vi "PreConfig.vi"(5 "Ruta de Transductores in":path, 7 "Ruta de Mediciones in":path, 8 "error in (no error)":errorcluster, 10 "Transductores":string[][](array[string]), 11 "Medidas":string[][](array[string])) -> (0 "error out":errorcluster, 2 "Transductores":string[][](table), 3 "Mediciones":string[][](array[string]), 4 "Ruta de Transductores Out":path, 6 "Ruta de Mediciones Out":path)   [LabVIEW 2014, in "ConfigProg.lvlib"]
doc: "Carga las Mediciones y los Transducotres."
uses:
  <vilib>/Utility/miscctls.llb/LVPointTypeDef.ctl
  <vilib>/Utility/file.llb/Read From Spreadsheet File (string).vi
  ConfigProg.lvlib
panel:
  in  "Cancel":bool
  in  "Save":bool
  in  "Ruta de Mediciones":path caption="Ruta de Mediciones:"
  in  "Ruta de Transductores":path caption="Ruta de Transductores:"
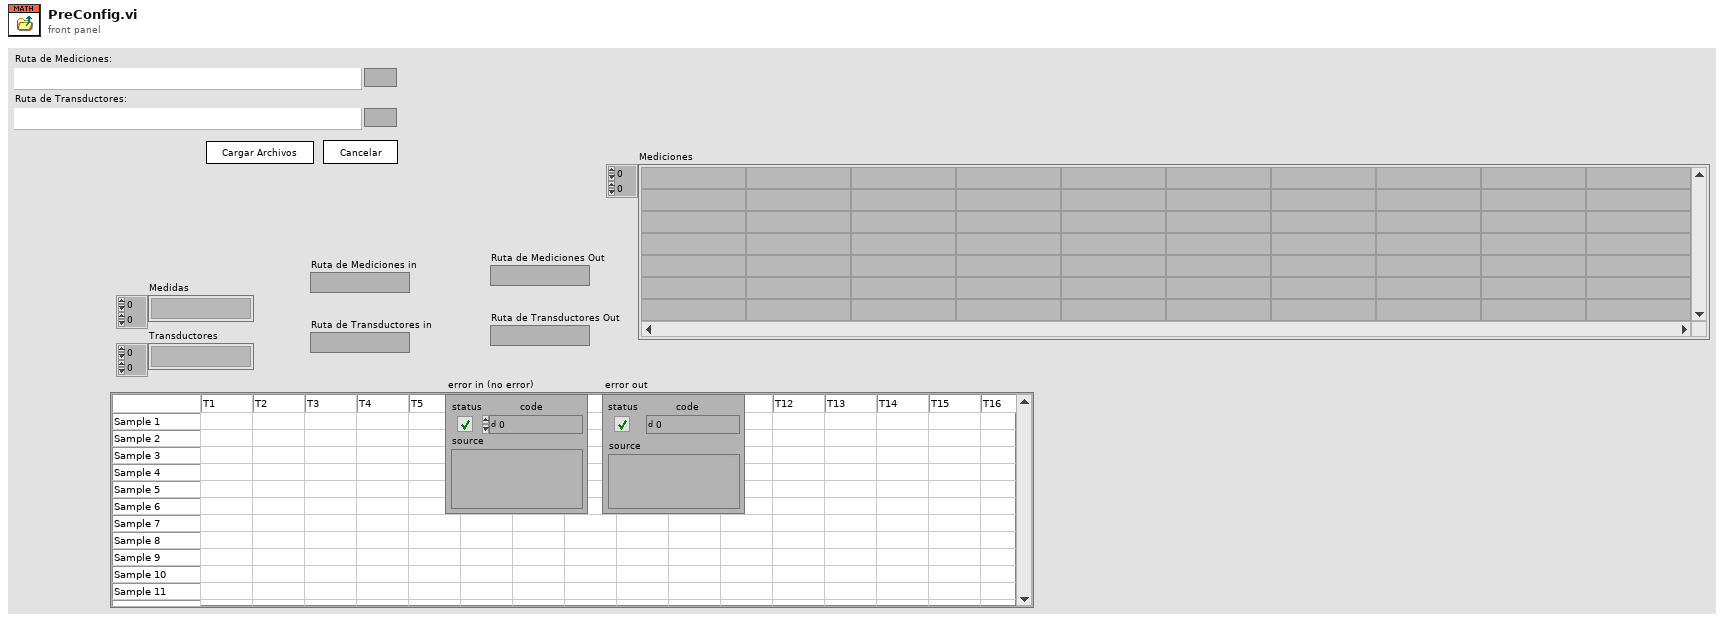
[diagram p1: front panel]
types:
  T1 = typedef "LVPointTypeDef.ctl" = cluster{"Horizontal":i16, "Vertical":i16}
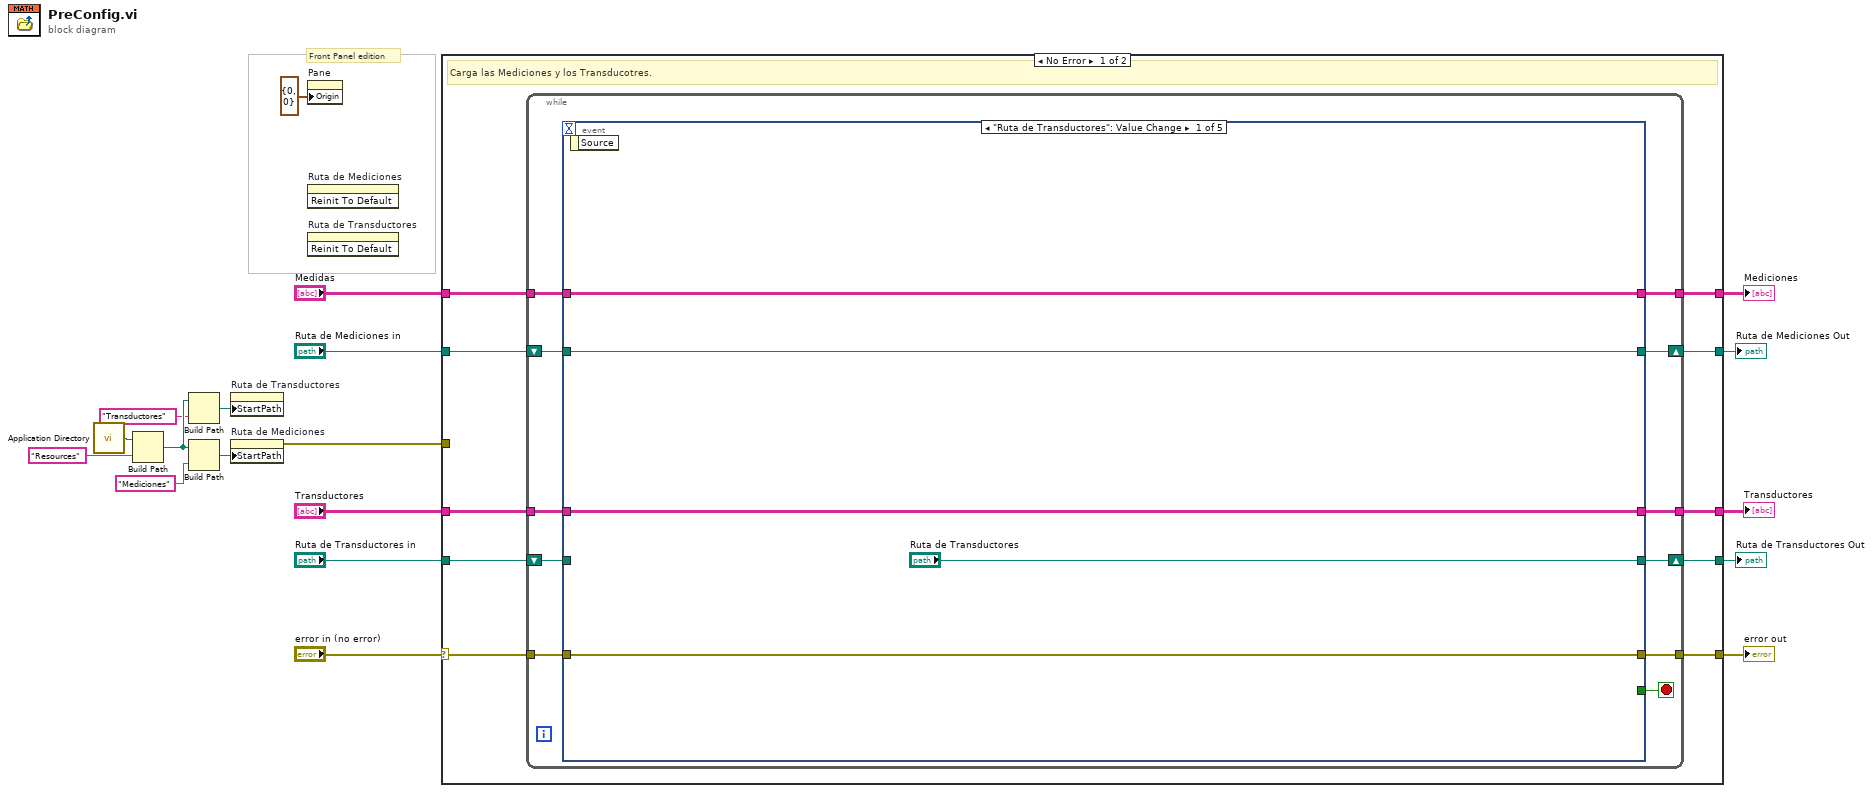
[diagram p0: block diagram]
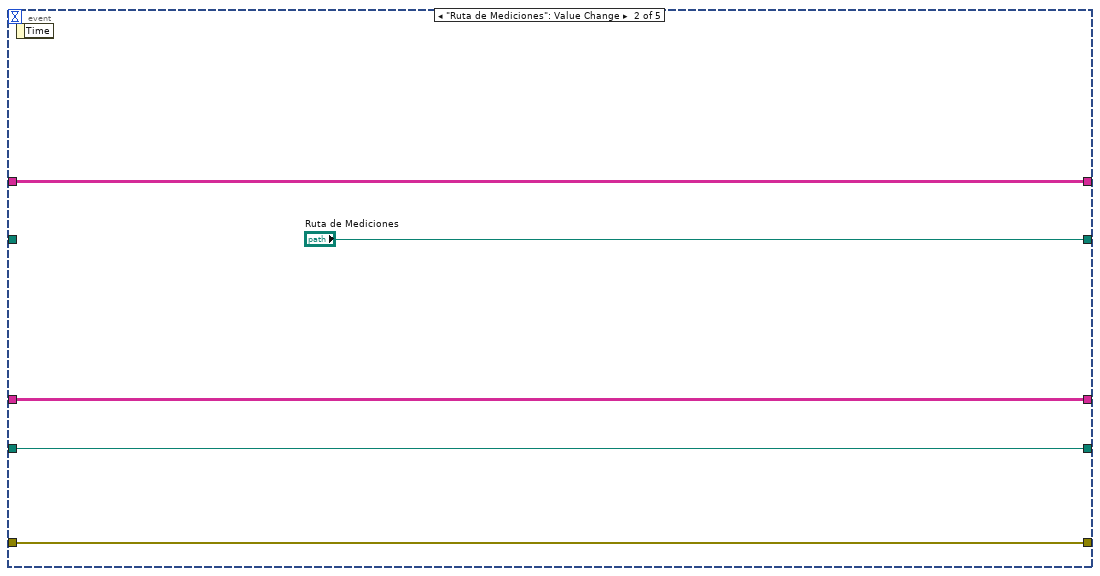
[diagram p2: hidden frame]
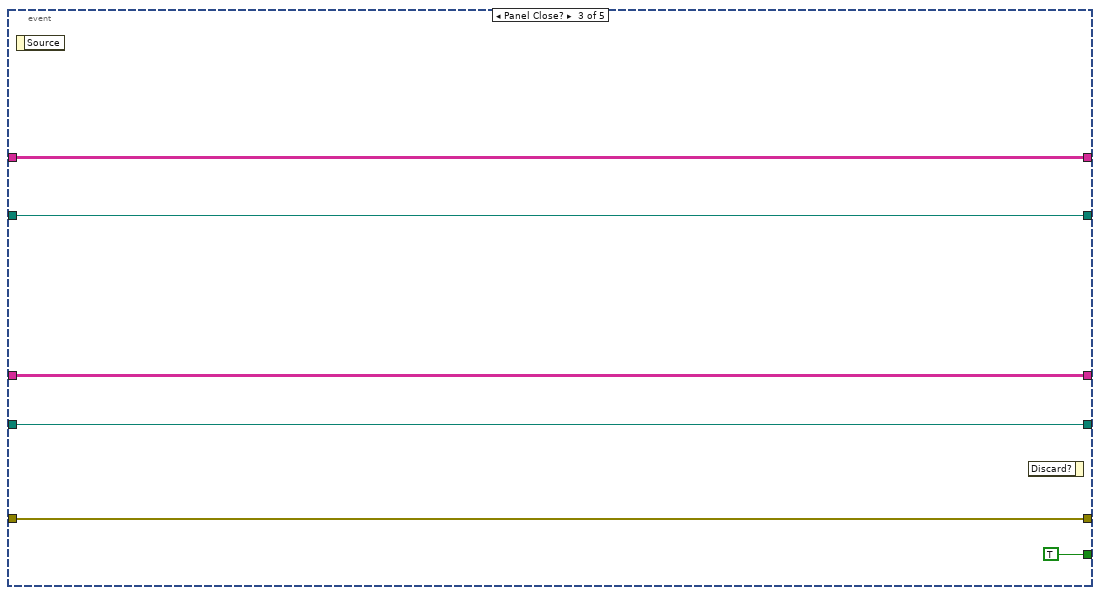
[diagram p3: hidden frame]
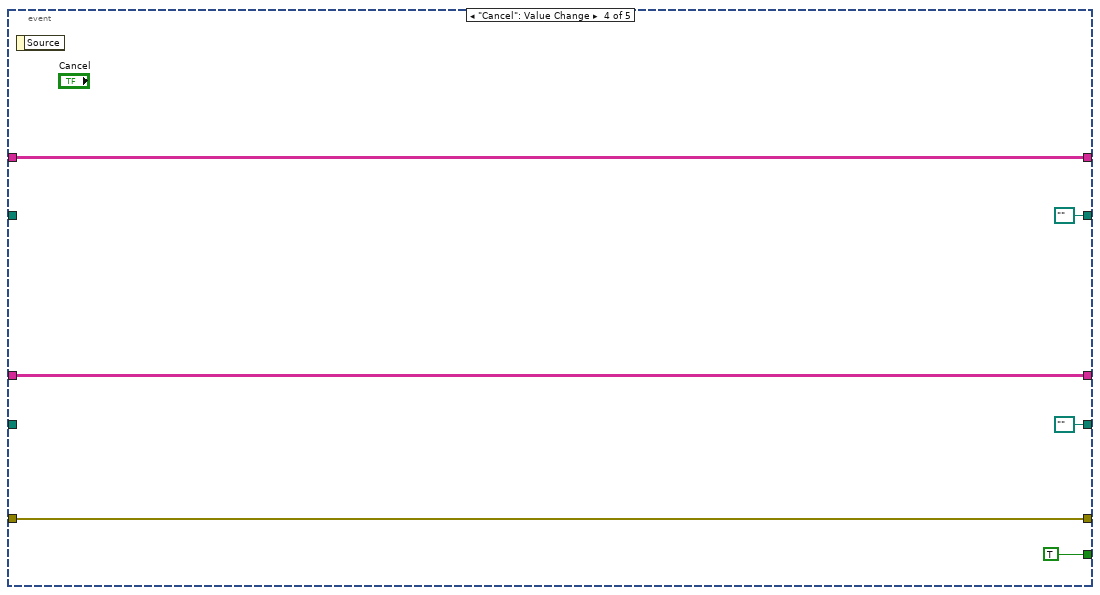
[diagram p4: hidden frame]
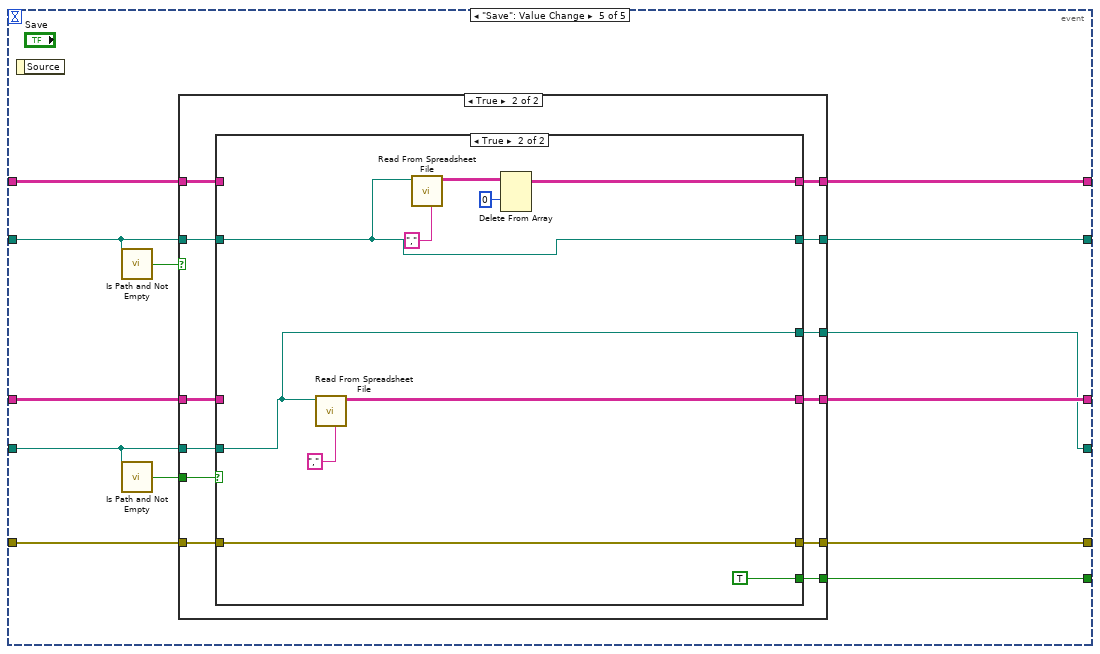
[diagram p5: hidden frame]
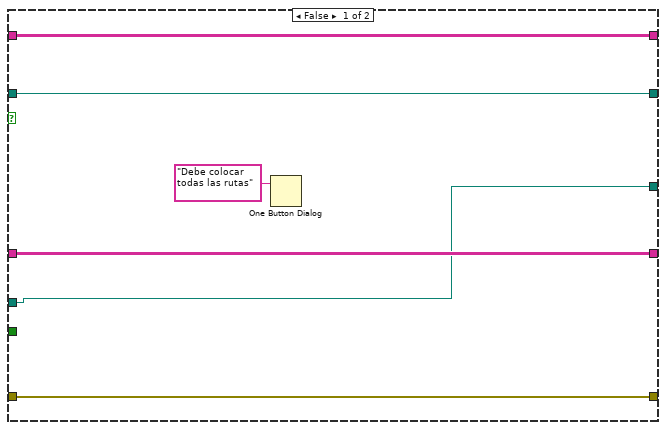
[diagram p6: hidden frame]
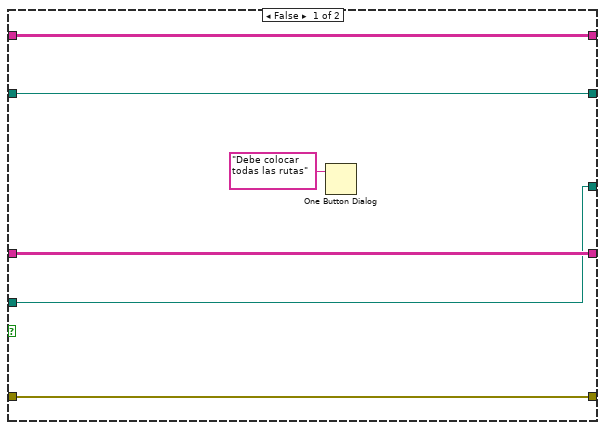
[diagram p7: hidden frame]
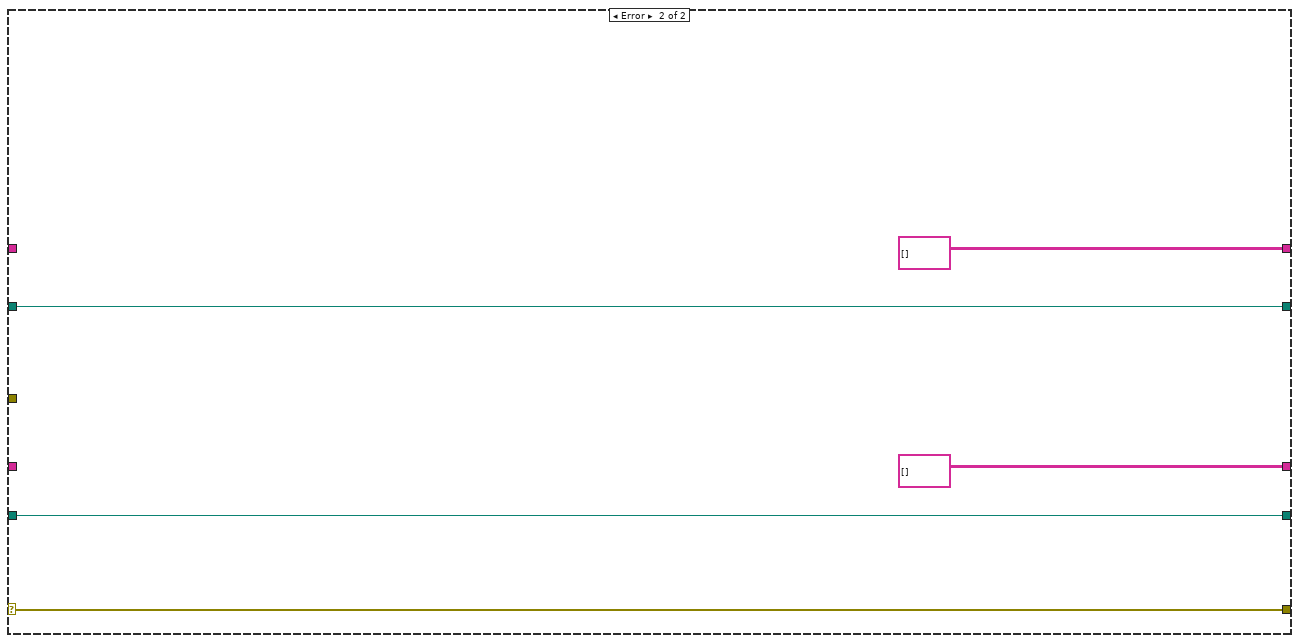
[diagram p8: hidden frame]
diagram:
  # "Front Panel edition"
  n1 = call <vilib>:"Application Directory.vi"() -> ("Application Directory"=w7:path)
  n2 = Build Path(base path=w7, name or relative path="Resources") -> (appended path=w6:path)
  n3 = Build Path(base path=w6, name or relative path="Transductores") -> (appended path=w3:path)
  n4 = Build Path(base path=w6, name or relative path="Mediciones") -> (appended path=w2:path)
  n5 = property on="Ruta de Transductores" class="Path"("StartPath"=w3) -> ()  [unwired: 2 in, 2 out]
  n6 = property on="Ruta de Mediciones" class="Path"("StartPath"=w2) -> (error out=w1:errorcluster)  [unwired: 2 in, 1 out]
  n7 = property on="Pane" class="Pane"("Origin"=T1 {"Horizontal"=0, "Vertical"=0}) -> ()  [unwired: 2 in, 2 out]
  n8 = invoke on="Ruta de Mediciones" class="Path" method="Reinit To Default"() -> ()  [unwired: 3 in, 3 out]
  n9 = invoke on="Ruta de Transductores" class="Path" method="Reinit To Default"() -> ()  [unwired: 3 in, 3 out]
  n10 = case shown="No Error" "error in (no error)" {
    selector: "error in (no error)" -> [w28 w114]
    tunnel: [w29 w114] -> w18
    tunnel: [w26 string[][] []] -> w16
    tunnel: [w27 string[][] []] -> w15
    tunnel: "Medidas" -> [w25 _]
    tunnel: "Transductores" -> [w24 _]
    tunnel: [w23 w111] -> w12
    tunnel: [w22 w110] -> w11
    tunnel: "Ruta de Mediciones in" -> [w21 w111]
    tunnel: "Ruta de Transductores in" -> [w20 w110]
    tunnel: w1 -> [_ _]
    frame No Error {
      # "Carga las Mediciones y los Transducotres."
      n11 = while {
        tunnel: w28 -> [w39]
        tunnel: [w40] -> w29
        shift-right: [w35] -> w22
        shift-left: w20 -> [w33]
        tunnel: [w34] -> w26
        shift-right: [w31] -> w23
        shift-left: w21 -> [w32]
        tunnel: w25 -> [w36]
        tunnel: [w38] -> w27
        tunnel: w24 -> [w30]
        stop <- w37 stop-if-true
        n12 = event shown="[0] \"Ruta de Transductores\": Value Change" {
          selector: _ -> [_ _ _ _ _]
          dyn-events: _ -> [_ _ _ _ _]
          timeout: _ -> [_ _ _ _ _]
          tunnel: [w41 w46 w51 w59 w75] -> w34
          tunnel: [w43 w50 w55 w61 w70] -> w40
          tunnel: w39 -> [w43 w50 w55 w61 w74]
          tunnel: [w45 w47 w52 w60 w73] -> w38
          tunnel: [_ _ TRUE ("Discard?") TRUE ("Discard?") w65] -> w37
          tunnel: w36 -> [w45 w47 w52 w60 w66]
          tunnel: ["Ruta de Transductores" w49 w53 path "" ("Ruta de Transductores in") w64] -> w35
          tunnel: w33 -> [_ w49 w53 _ w71]
          tunnel: w32 -> [w42 _ w54 _ w72]
          tunnel: [w42 "Ruta de Mediciones" w54 path "" ("Ruta de Mediciones in") w63] -> w31
          tunnel: w30 -> [w41 w46 w51 w59 w67]
          event "Ruta de Transductores": Value Change {
            n13 = event-data() -> ()  [unwired: 1 in, 1 out]
          }
          event "Ruta de Mediciones": Value Change {
            n14 = event-data() -> ()  [unwired: 1 in, 1 out]
          }
          event Panel Close? {
            n15 = event-data() -> ()  [unwired: 1 in, 1 out]
            n16 = event-data() -> ()  [unwired: 2 in, 1 out]
          }
          event "Cancel": Value Change {
            n17 = event-data() -> ()  [unwired: 1 in, 1 out]
          }
          event "Save": Value Change {
            n18 = event-data() -> ()  [unwired: 1 in, 1 out]
            n19 = call <vilib>:"Is Path and Not Empty.vi"("path"=w72) -> ("Is Path and Not Empty?"=w69:bool)  [unwired: 4 in]
            n20 = call <vilib>:"Is Path and Not Empty.vi"("path"=w71) -> ("Is Path and Not Empty?"=w68:bool)  [unwired: 4 in]
            n21 = case shown="True" w69 {
              tunnel: [w80 w93] -> w75
              tunnel: w74 -> [w78 w92]
              tunnel: [w79 w91] -> w73
              tunnel: w72 -> [w77 w90]
              tunnel: w71 -> [w76 w89]
              tunnel: [w78 w88] -> w70
              tunnel: w68 -> [_ w87]
              tunnel: w67 -> [w80 w86]
              tunnel: w66 -> [w79 w85]
              tunnel: [_ w84] -> w65
              tunnel: [w76 w83] -> w64
              tunnel: [w77 w82] -> w63
              frame False {
                n22 = One Button Dialog(message="Debe colocar todas las rutas") -> ()  [unwired: 1 in, 1 out]
              }
              frame True {
                n23 = case shown="True" w87 {
                  tunnel: [w98 w101] -> w93
                  tunnel: w92 -> [w96 w100]
                  tunnel: [w97 w105] -> w91
                  tunnel: w90 -> [w95 w102]
                  tunnel: w89 -> [w94 w103]
                  tunnel: [w96 w100] -> w88
                  tunnel: w86 -> [w98 _]
                  tunnel: w85 -> [w97 _]
                  tunnel: [_ TRUE ("Discard?")] -> w84
                  tunnel: [w94 w103] -> w83
                  tunnel: [w95 w102] -> w82
                  frame False {
                    n24 = One Button Dialog(message="Debe colocar todas las rutas") -> ()  [unwired: 1 in, 1 out]
                  }
                  frame True {
                    n25 = call-poly <vilib>:"Read From Spreadsheet File.vi"("delimiter (\\t)"="," ("delimiter (\\t)"), "file path (dialog if empty)"=w103) -> ("all rows"=w101:string[][])  [unwired: 5 in, 4 out]
                    n26 = call-poly <vilib>:"Read From Spreadsheet File.vi"("delimiter (\\t)"="," ("delimiter (\\t)"), "file path (dialog if empty)"=w102) -> ("all rows"=w106:string[][])  [unwired: 5 in, 4 out]
                    n27 = Delete From Array(array=w106, index (row)=0 ("index")) -> (array with subset deleted=w105:string[][])  [unwired: 2 in, 1 out]
                  }
                }
              }
            }
          }
        }
      }
    }
    frame Error {
    }
  }
  "error out" <- w18
  "Transductores" <- w16
  "Mediciones" <- w15
  "Ruta de Mediciones Out" <- w12
  "Ruta de Transductores Out" <- w11
